vi "Read any file waveform.vi"(4 "(BINARY) 2D number of rows":i32, 6 "(BINARY) 2D number of columns/1D count (all as 1D: -1)":i32=1, 7 "tdms file in":refnum<k34>, 8 "error in":errorcluster, 9 "Data File Type":T2(ring), 10 "Data window":T1={"Start"=0, "Length"=500000, "Channel numbers"=[0], "Channel names"=["Bdot", "Freq"], "Group name"="Untitled"}, 11 "Input file path":path) -> (0 "error out":errorcluster, 1 "1st channel length":u64, 2 "Data out":waveform(dbl)[](array[waveform]), 3 "Actual input file path":path, 5 "tdms file out":refnum<k34>)   [LabVIEW 2015]
panel:
  out "Header":string
  # "OR"
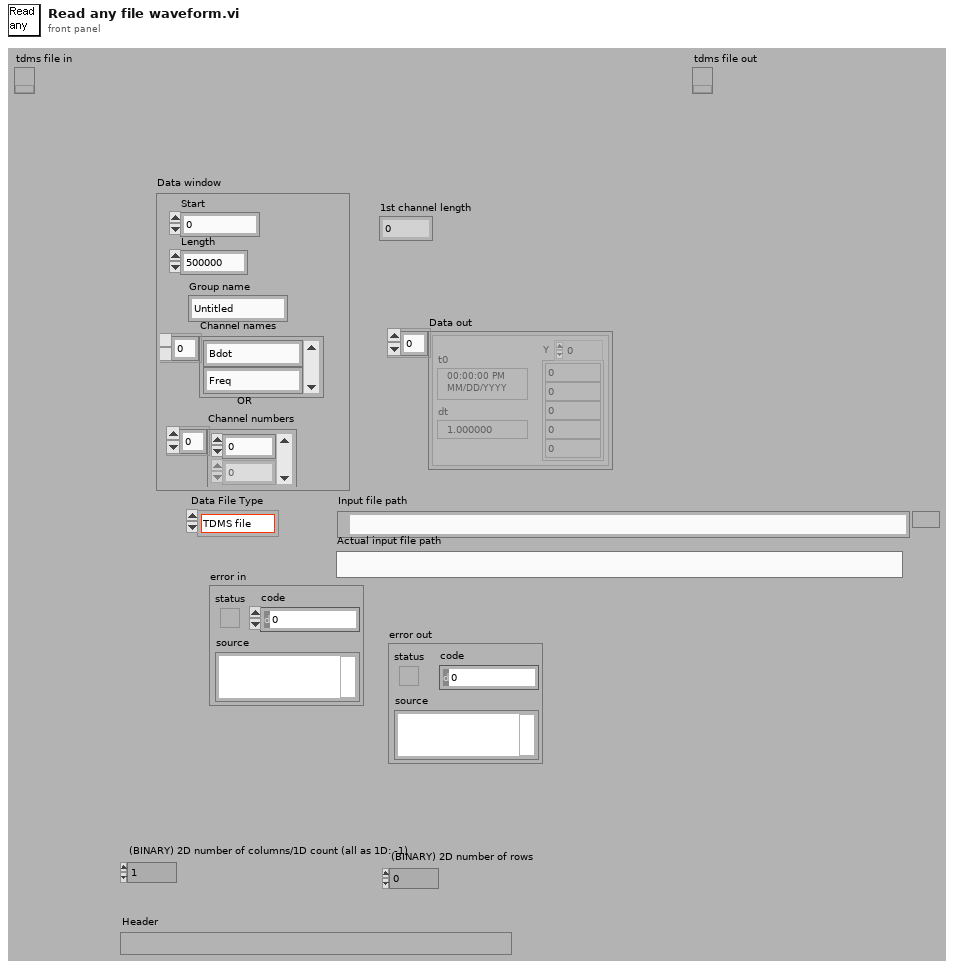
[diagram p1: front panel]
types:
  T1 = cluster{"Start":i64, "Length":i32, "Channel numbers":i64[], "Channel names":string[], "Group name":string}
  T2 = enum16{"TDMS file", "Tektronics ISF", "BinF file", "ASCII File", "BinH File", "BinW File", "BINARY File"}
  T3 = enum16{"open", "open or create", "create or replace", "create", "open (read-only)"}
  T4 = cluster{"Version":i16, "Data Representation":enum16{"Undefined", "I8", "I16", "I32", "I64", "U8", "U16", "U32", "U64", "SGL", "DBL", "EXT"}, "# columns (samples per channel)":i64, "# rows (channels)":i64, "# pre-trigger samples":i64, "Sample rate":dbl, "ADC offset":dbl, "Scale factor":dbl}
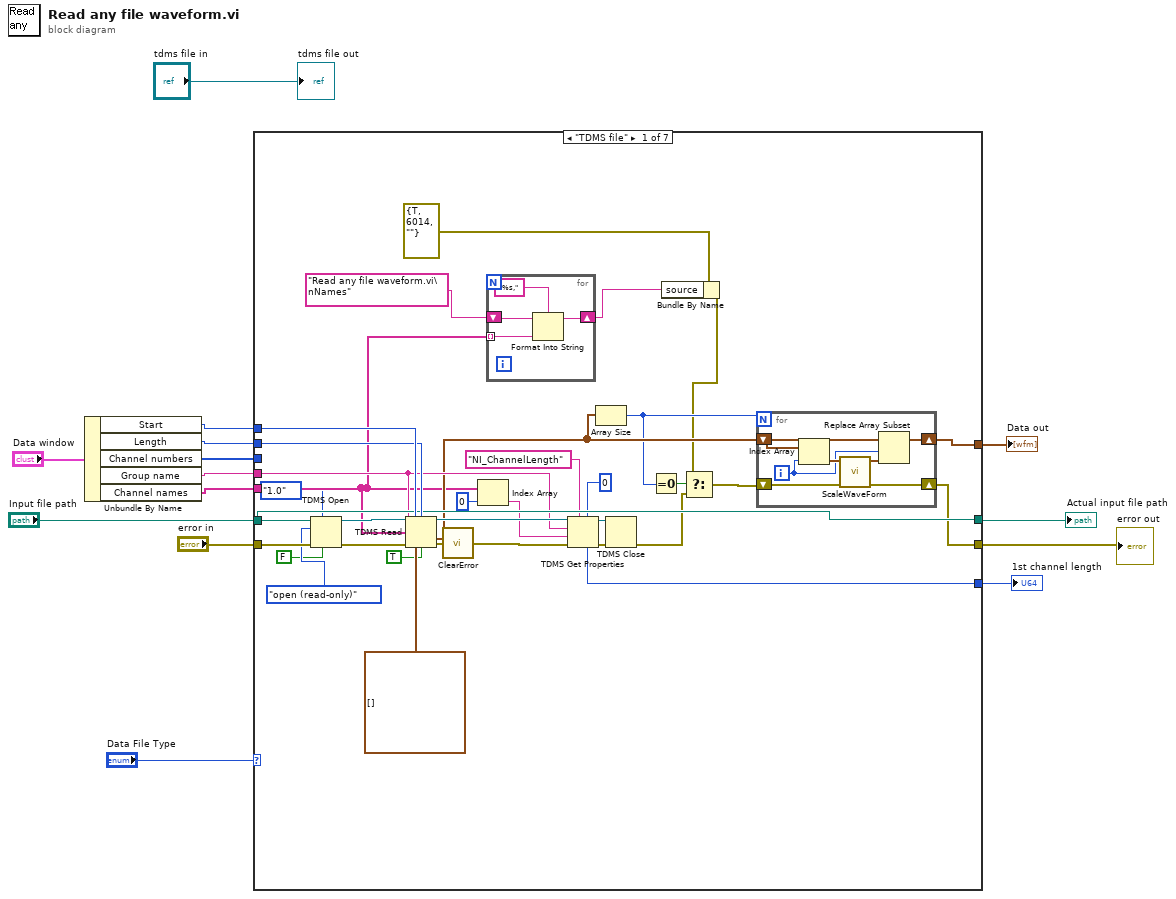
[diagram p0: block diagram]
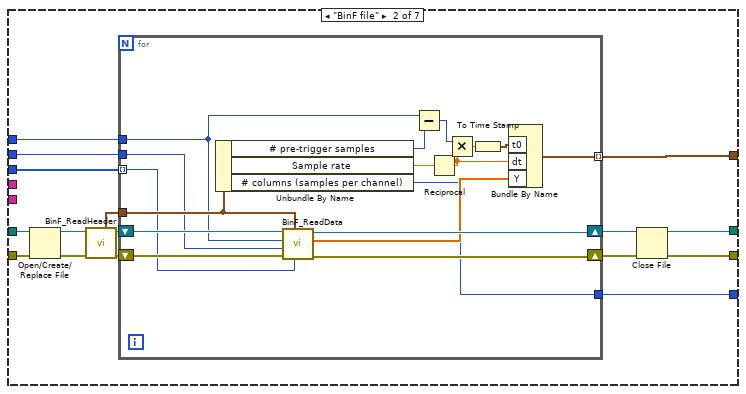
[diagram p2: hidden frame]
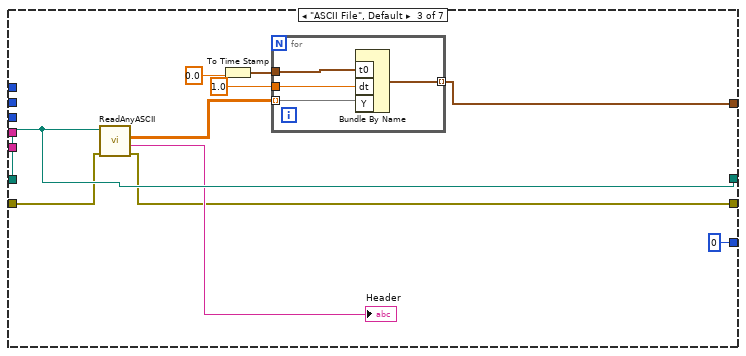
[diagram p3: hidden frame]
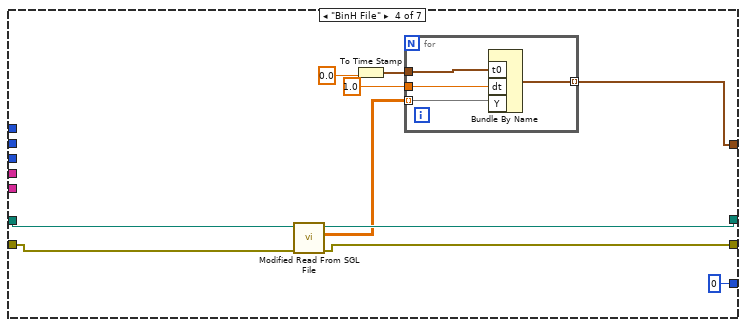
[diagram p4: hidden frame]
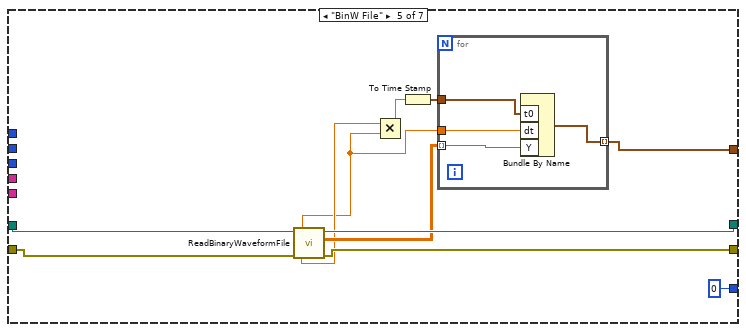
[diagram p5: hidden frame]
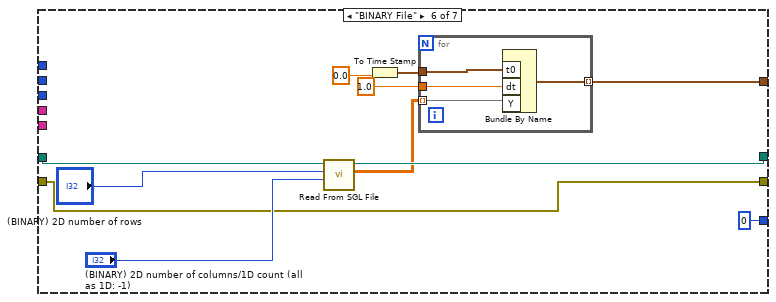
[diagram p6: hidden frame]
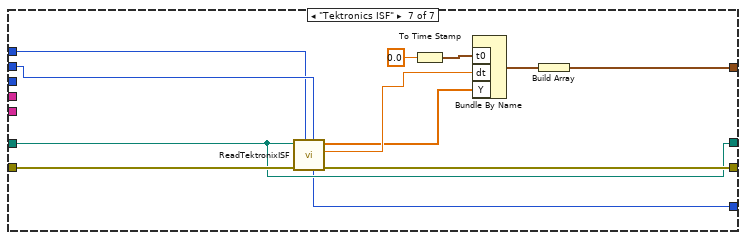
[diagram p7: hidden frame]
diagram:
  n1 = Unbundle By Name("Data window") -> ("Start"=w9:i64, "Length"=w8:i32, "Channel numbers"=w10:i64[], "Group name"=w4:string, "Channel names"=w6:string[])
  n2 = case shown="\"TDMS file\"" "Data File Type" {
    tunnel: "Input file path" -> [w41 w73 w96 w116 w131 w146 w153]
    tunnel: [w41 w65 w96 w115 w130 w145 w153] -> w12
    tunnel: "error in" -> [w48 w72 w94 w114 w129 w138 w156]
    tunnel: [w30 w66 w93 w113 w128 w138 w155] -> w2
    tunnel: w10 -> [_ w64 _ _ _ _ _]
    tunnel: w9 -> [w44 w63 _ _ _ _ w157]
    tunnel: w8 -> [w43 w62 _ _ _ _ w158]
    tunnel: [w31 w61 w99 w109 w127 w142 w152] -> w7
    tunnel: w6 -> [w19 _ _ _ _ _ _]
    tunnel: [w33 w60 u64 0 ("# columns (samples per channel)") u64 0 ("# columns (samples per channel)") u64 0 ("# columns (samples per channel)") u64 0 ("# columns (samples per channel)") w151] -> w5
    tunnel: w4 -> [w32 _ _ _ _ _ _]
    frame "TDMS file" {
      n3 = TDMS Open(6:FALSE ("disable buffering (T)"), 7:enum16{"1.0", "2.0"}."1.0" ("file format version (2.0)"), 8:w48, 10:T3."open (read-only)" ("operation (0:open)"), 11:w41) -> (0:w46:errorcluster, 3:w47:refnum<k34>)  [unwired: 2 in]
      n4 = TDMS Read(0:w47, 1:w44, 2:w43, 5:w32, 7:w19, 11:w46, 12:waveform(dbl)[] [], 13:TRUE ("return channels in file order? (F)")) -> (4:w39:refnum<k34>, 10:w29:waveform(dbl)[], 15:w18:errorcluster)  [unwired: 3 out]
      n5 = call <vilib>:"ClearError.vi"("error in (no error)"=w18) -> ("error out"=w42:errorcluster)
      n6 = Index Array(array=w19, index=0) -> (element=w36:string)
      n7 = for {
        shift-right: [w50] -> w20
        shift-left: "Read any file waveform.vi\nNames" -> [w52]
        tunnel: w19 -> [w49] mode=indexing
        n8 = Format Into String(format string=" %s,", initial string=w52, w49) -> (resulting string=w50:string)  [unwired: 1 in, 1 out]
      }
      n9 = TDMS Get Properties(5:u64 0, 7:"NI_ChannelLength" ("property name"), 8:w42, 9:w36, 10:w32, 11:w39) -> (0:w40:errorcluster, 3:w38:refnum<k34>, 4:w33:u64)  [unwired: 3 out]
      n10 = Array Size(array=w29) -> (size(s)=w24:i32)
      n11 = TDMS Close(8:w40, 11:w38) -> (0:w26:errorcluster)  [unwired: 1 out]
      n12 = Equal To 0?(x=w24) -> (x = 0?=w25:bool)
      n13 = Bundle By Name(cluster=errorcluster {"status"=TRUE, "code"=6014, "source"=""} ("t"), "source"=w20) -> (w22:errorcluster)
      n14 = Select(t=w22, s=w25, f=w26) -> (s? t:f=w27:errorcluster)
      n15 = for {
        N: w24 -> [_]
        shift-right: [w58] -> w31
        shift-left: w29 -> [w57]
        shift-right: [w54] -> w30
        shift-left: w27 -> [w55]
        i -> [w53]
        n16 = Index Array(array=w57, index=w53) -> (element=w59:waveform(dbl))
        n17 = call "ScaleWaveForm.vi"("error in (no error)"=w55, "Waveform"=w59) -> ("error out"=w54:errorcluster, "Scaled Waveform"=w56:waveform(sgl))  [unwired: 8 out]
        n18 = Replace Array Subset(array=w57, new element=w56, index=w53) -> (w58:waveform(dbl)[])
      }
    }
    frame "BinF file" {
      n19 = Open/Create/Replace File(file path (use dialog)=w73, error in=w72) -> (refnum out=w74:refnum<file>, error out=w75:errorcluster)  [unwired: 5 out]
      n20 = call "BinF_ReadHeader.vi"("error in"=w75, "refnum"=w74) -> ("error out"=w71:errorcluster, "refnum out"=w70:refnum<file>, "BinF File Settings"=w69:T4)  [unwired: 7 out]
      n21 = for {
        shift-right: [w91] -> w68
        shift-left: w71 -> [w92]
        shift-right: [w89] -> w67
        shift-left: w70 -> [w90]
        tunnel: w69 -> [w82]
        tunnel: w64 -> [w81] mode=indexing
        tunnel: w63 -> [w79]
        tunnel: w62 -> [w80]
        tunnel: [w77] -> w61 mode=indexing
        tunnel: [w76] -> w60
        n22 = Unbundle By Name(w82) -> ("# pre-trigger samples"=w86:i64, "Sample rate"=w84:dbl, "# columns (samples per channel)"=w76:i64)
        n23 = call "BinF_ReadData.vi"("Channel number"=w81, "BinF File Settings"=w82, "error in"=w92, "Length"=w80, "Start"=w79, "refnum"=w90) -> ("error out"=w91:errorcluster, "Channel Data"=w78:sgl[], "refnum out"=w89:refnum<file>)  [unwired: 3 out]
        n24 = Subtract(x=w79, y=w86) -> (x-y=w87:i64)
        n25 = Reciprocal(x=w84) -> (1/x=w85:dbl)
        n26 = Multiply(x=w87, y=w85) -> (x*y=w88:dbl)
        n27 = To Time Stamp(1:w88) -> (0:w83:timestamp)
        n28 = Bundle By Name("t0"=w83, "dt"=w85, "Y"=w78) -> (w77:waveform(sgl))  [unwired: 1 out]
      }
      n29 = Close File(refnum=w67, error in=w68) -> (path=w65:path, error out=w66:errorcluster)
    }
    frame "ASCII File", Default {
      n30 = call "ReadAnyASCII.vi"("error in (no error)"=w94, "file path (dialog if empty)"=w96) -> ("error out"=w93:errorcluster, "Header text"=→"Header":string, "all rows"=w98:dbl[][])  [unwired: 2 in, 5 out]
      n31 = To Time Stamp(1:0.0) -> (0:w101:timestamp)
      n32 = for {
        tunnel: w98 -> [w106] mode=indexing
        tunnel: [w105] -> w99 mode=indexing
        tunnel: w101 -> [w104]
        tunnel: 1.0 -> [w103]
        n33 = Bundle By Name("t0"=w104, "dt"=w103, "Y"=w106) -> (w105:waveform(dbl))  [unwired: 1 out]
      }
    }
    frame "BinH File" {
      n34 = call "Modified Read From SGL File.vi"("error in (no error)"=w114, "file path (dialog if empty)"=w116) -> ("error out"=w113:errorcluster, "2D array"=w108:sgl[][], "new file path (Not A Path if cancelled)"=w115:path)  [unwired: 1 in, 6 out]
      n35 = To Time Stamp(1:0.0) -> (0:w111:timestamp)
      n36 = for {
        tunnel: w108 -> [w120] mode=indexing
        tunnel: [w119] -> w109 mode=indexing
        tunnel: w111 -> [w118]
        tunnel: 1.0 -> [w117]
        n37 = Bundle By Name("t0"=w118, "dt"=w117, "Y"=w120) -> (w119:waveform(sgl))  [unwired: 1 out]
      }
    }
    frame "BinW File" {
      n38 = call "ReadBinaryWaveformFile.vi"("error in (no error)"=w129, "file path (dialog if empty)"=w131) -> ("error out"=w128:errorcluster, "2D array"=w126:sgl[][], "new file path (Not A Path if cancelled)"=w130:path, "Time base"=w125:dbl, "Delay, points"=w122:dbl)  [unwired: 1 in, 4 out]
      n39 = Multiply(x=w125, y=w122) -> (x*y=w124:dbl)
      n40 = To Time Stamp(1:w124) -> (0:w123:timestamp)
      n41 = for {
        tunnel: w126 -> [w134] mode=indexing
        tunnel: [w135] -> w127 mode=indexing
        tunnel: w123 -> [w133]
        tunnel: w122 -> [w132]
        n42 = Bundle By Name("t0"=w133, "dt"=w132, "Y"=w134) -> (w135:waveform(sgl))  [unwired: 1 out]
      }
    }
    frame "BINARY File" {
      n43 = call <vilib>:"Read From SGL File.vi"("2D number of columns/1D count (all as 1D: -1)"="(BINARY) 2D number of columns/1D count (all as 1D: -1)", "2D number of rows"="(BINARY) 2D number of rows", "file path (dialog if empty)"=w146) -> ("2D array"=w143:sgl[][], "new file path (Not A Path if cancelled)"=w145:path)  [unwired: 7 out]
      n44 = To Time Stamp(1:0.0) -> (0:w140:timestamp)
      n45 = for {
        tunnel: w143 -> [w150] mode=indexing
        tunnel: [w149] -> w142 mode=indexing
        tunnel: w140 -> [w148]
        tunnel: 1.0 -> [w147]
        n46 = Bundle By Name("t0"=w148, "dt"=w147, "Y"=w150) -> (w149:waveform(sgl))  [unwired: 1 out]
      }
    }
    frame "Tektronics ISF" {
      n47 = call "ReadTektronixISF.vi"("Length"=w158, "Start"=w157, "error in (no error)"=w156, "Path"=w153) -> ("error out"=w155:errorcluster, "dt"=w162:dbl, "Data"=w154:dbl[], "Total number of points"=w151:u64)  [unwired: 4 out]
      n48 = To Time Stamp(1:0.0) -> (0:w159:timestamp)
      n49 = Bundle By Name("t0"=w159, "dt"=w162, "Y"=w154) -> (w161:waveform(dbl))  [unwired: 1 out]
      n50 = Build Array(w161) -> (w152:waveform(dbl)[])
    }
  }
  "Actual input file path" <- w12
  "error out" <- w2
  "Data out" <- w7
  "1st channel length" <- w5
  "tdms file out" <- "tdms file in"
